vi "MotorMain.vi"() -> ()   [LabVIEW 2011]
uses:
  Main/Motors/MotorConfigType.ctl
  Main/Motors/MotorPosType.ctl
  Main/Typedefs/XYf.ctl
  Main/Motors/MotorPosFlagsType.ctl
  Modules/PIMotorController/PI_Axis_list.ctl
  Modules/PIMotorController/PI_Axis.ctl
panel:
  out "Conn. \nAxes 2":string[](array[string])
  out "Conn. \nAxes":string[](array[string])
  out "All conn. axes":string[](array[string])
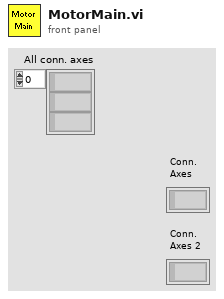
[diagram p1: front panel]
types:
  T1 = typedef "MotorConfigType.ctl" = cluster{"Offset":T2, "Maximum pos":T2, "Min limited?":T4, "Max limited?":T4, "Has velocity support":T4, "Default velocity":T2}
  T2 = typedef "MotorPosType.ctl" = cluster{"Magnet Z":dbl, "Magnet rotation":dbl, "Camera":T3, "Piezo XY":T3, "Piezo Z":dbl}
  T3 = typedef "XYf.ctl" = cluster{"X":sgl, "Y":sgl}
  T4 = typedef "MotorPosFlagsType.ctl" = cluster{"Magnet Z":bool, "Magnet rotation":bool, "Camera":cluster{"X":bool, "Y":bool}, "Piezo XY":cluster{"X":bool, "Y":bool}, "Piezo Z":bool}
  T5 = typedef "PI_Axis_list.ctl" = cluster{"Piezo X":T6, "Piezo Y":T6, "Piezo Z":T6, "Magnet Z":T6, "Magnet Rotation":T6, "Objective X":T6, "Objective Y":T6}
  T6 = typedef "PI_Axis.ctl" = cluster{"System #":i32, "Axis ID":string, "Multiplier":dbl}
  T7 = typedef "GCS_Interface.ctl" = cluster{"MOV":refnum<vi>, "VEL":refnum<vi>, "VEL?":refnum<vi>, "POS?":refnum<vi>, "TMX?":refnum<vi>, "#7 (Ready?)":refnum<vi>, "FPL":refnum<vi>, "FNL":refnum<vi>}
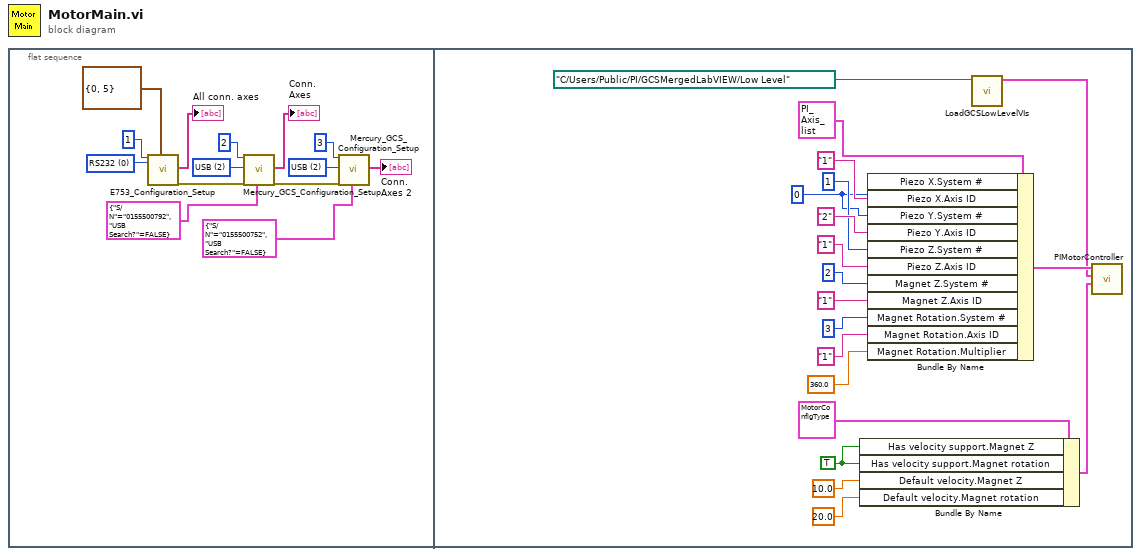
[diagram p0: block diagram]
diagram:
  n1 = flat-sequence {
    frame #0 {
      w2 = u16 0 items=["RS232", "TCP/IP", "USB"] ("Interface")
      w10 = u16 2 items=["RS232", "RS232 DaisyChain", "USB", "USB_DaisyChain"] ("Interface")
      w13 = u16 2 items=["RS232", "RS232 DaisyChain", "USB", "USB_DaisyChain"] ("Interface")
      n2 = call "E753_Configuration_Setup.vi"("System no."=1, "Interface"=w2, "RS232 settings"=cluster{"Portnumber":i32, "Baudrate":u16} {"Portnumber"=0, "Baudrate"=5}) -> ("Conn. \nAxis"=→"All conn. axes":string[], "error out"=w4:errorcluster)  [unwired: 11 in, 4 out]
      n3 = call "Mercury_GCS_Configuration_Setup.vi"("System no."=2, "Interface"=w13, "error in"=w4, "USB settings"=cluster{"S/N":string, "USB Search?":bool} {"S/N"="0155500792", "USB Search?"=FALSE}) -> ("Conn. \nAxes"=→"Conn. \nAxes":string[], "error out"=w5:errorcluster)  [unwired: 9 in, 5 out]
      n4 = call "Mercury_GCS_Configuration_Setup.vi"("System no."=3, "Interface"=w10, "error in"=w5, "USB settings"=cluster{"S/N":string, "USB Search?":bool} {"S/N"="0155500752", "USB Search?"=FALSE}) -> ("Conn. \nAxes"=→"Conn. \nAxes 2":string[])  [unwired: 9 in, 6 out]
    }
    frame #1 {
      w15 = 0 ("Piezo X.System #")
      w25 = TRUE ("Has velocity support.Magnet Z")
      n5 = Bundle By Name(cluster=T1 {"Offset"={"Magnet Z"=0.0, "Magnet rotation"=0.0, "Camera"={"X"=0.0, "Y"=0.0}, "Piezo XY"={"X"=0.0, "Y"=0.0}, "Piezo Z"=0.0}, "Maximum pos"={"Magnet Z"=0.0, "Magnet rotation"=0.0, "Camera"={"X"=0.0, "Y"=0.0}, "Piezo XY"={"X"=0.0, "Y"=0.0}, "Piezo Z"=0.0}, "Min limited?"={"Magnet Z"=FALSE, "Magnet rotation"=FALSE, "Camera"={"X"=FALSE, "Y"=FALSE}, "Piezo XY"={"X"=FALSE, "Y"=FALSE}, "Piezo Z"=FALSE}, "Max limited?"={"Magnet Z"=FALSE, "Magnet rotation"=FALSE, "Camera"={"X"=FALSE, "Y"=FALSE}, "Piezo XY"={"X"=FALSE, "Y"=FALSE}, "Piezo Z"=FALSE}, "Has velocity support"={"Magnet Z"=TRUE, "Magnet rotation"=TRUE, "Camera"={"X"=FALSE, "Y"=FALSE}, "Piezo XY"={"X"=FALSE, "Y"=FALSE}, "Piezo Z"=FALSE}, "Default velocity"={"Magnet Z"=0.0, "Magnet rotation"=0.0, "Camera"={"X"=0.0, "Y"=0.0}, "Piezo XY"={"X"=0.0, "Y"=0.0}, "Piezo Z"=0.0}} ("MotorConfig"), "Has velocity support.Magnet Z"=w25, "Has velocity support.Magnet rotation"=w25, "Default velocity.Magnet Z"=10.0, "Default velocity.Magnet rotation"=20.0) -> (w22:T1)
      n6 = Bundle By Name(cluster=T5 {"Piezo X"={"System #"=0, "Axis ID"="", "Multiplier"=1.0}, "Piezo Y"={"System #"=0, "Axis ID"="", "Multiplier"=1.0}, "Piezo Z"={"System #"=0, "Axis ID"="", "Multiplier"=1.0}, "Magnet Z"={"System #"=0, "Axis ID"="", "Multiplier"=1.0}, "Magnet Rotation"={"System #"=0, "Axis ID"="", "Multiplier"=1.0}, "Objective X"={"System #"=0, "Axis ID"="", "Multiplier"=1.0}, "Objective Y"={"System #"=0, "Axis ID"="", "Multiplier"=1.0}} ("PI Axis config"), "Piezo X.System #"=w15, "Piezo X.Axis ID"="1", "Piezo Y.System #"=w15, "Piezo Y.Axis ID"="2", "Piezo Z.System #"=1 ("Piezo X.System #"), "Piezo Z.Axis ID"="1", "Magnet Z.System #"=2, "Magnet Z.Axis ID"="1", "Magnet Rotation.System #"=3, "Magnet Rotation.Axis ID"="1", "Magnet Rotation.Multiplier"=360.0) -> (w32:T5)
      n7 = call "LoadGCSLowLevelVIs.vi"("GCS Merged Drivers Low-Level Path"=path "C:/Users/Public/PI/GCSMergedLabVIEW/Low Level") -> ("PI GCS Function\nReferences"=w28:T7)  [unwired: 10 in]
      n8 = call "PIMotorController.vi"("MotorConfig"=w22, "PI GCS Function\nReferences"=w28, "PI Axis config"=w32) -> ()  [unwired: 9 in]
    }
  }
